vi "LVClass_Camera get Parameter Int.vi"(0 "Camera in":refnum<class "Camera.lvclass">, 7 "parameter_name":string, 11 "error in (no error)":errorcluster) -> (4 "Camera out":refnum<class "Camera.lvclass">, 8 "value":i32, 15 "error out":errorcluster)   [LabVIEW 2020, in "Camera.lvclass"]
doc: "Camera parameter getter for parameter of type E_TYPE_INT.\n\n<B>CameraIn</B> : Camera object.\n<B>CameraOut</B> : Camera object.\n<B>parameter_name</B> : Name of the parameter.\n<B>value</B> : Value of the parameter."
uses:
  Camera.lvclass
  Camera.lvclass/Camera.ctl
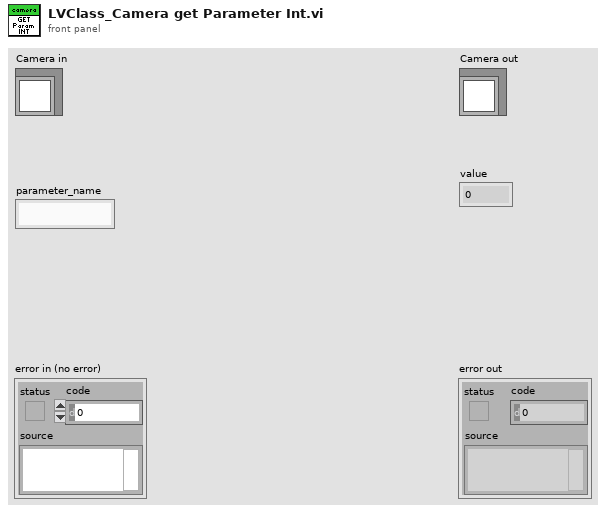
[diagram p1: front panel]
types:
  T1 = typedef "ClassID.ctl" = i64
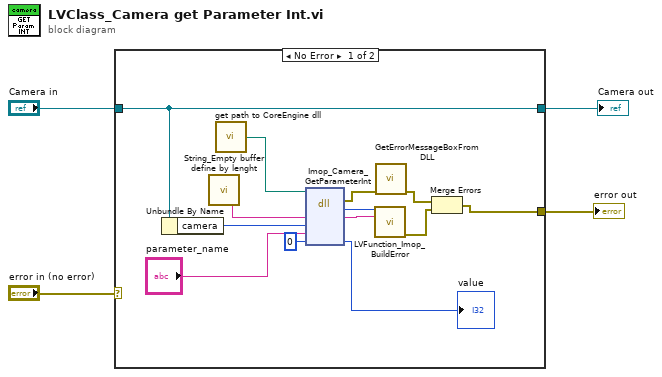
[diagram p0: block diagram]
diagram:
  n1 = case shown="No Error" "error in (no error)" {
    selector: "error in (no error)" -> [_ w19]
    tunnel: [w5 w19] -> w3
    tunnel: [w13 w18] -> w1
    tunnel: "Camera in" -> [w13 w18]
    frame No Error {
      n2 = Unbundle By Name(w13) -> ("camera"=w14:T1)
      n3 = call "String_Empty buffer define by lenght.vi"() -> ("Empty buffer"=w17:string)  [unwired: 1 in]
      n4 = call "get path to CoreEngine dll.vi"() -> ("path to c_interface_vc100.dll"=w12:path)  [unwired: 12 in, 3 out]
      n5 = dll-call lib="D:/2_trunk/Soft_haso/ImOpCoreEngine4_LV2011/DLLs/ImopEngine4_vc100.dll" fn="Imop_Camera_GetParameterInt"(path in=w12, "message"=w17, "camera"=w14, "parameter_name"="parameter_name", "value"=u32 0) -> (error out=w11:errorcluster, "return type"=w16:i32, "message"=w15:string, "value"=→"value":i32)  [unwired: 4 in, 1 out]
      n6 = call "LVFunction_Imop_BuildError.vi"("code"=w16, "String to Prepend to source (\"\")"=w15) -> ("error out"=w6:errorcluster)  [unwired: 13 in]
      n7 = call "GetErrorMessageBoxFromDLL.vi"("error IN"=w11) -> ("error OUT"=w7:errorcluster)  [unwired: 10 in]
      n8 = Merge Errors(w7, w6) -> (w5:errorcluster)
    }
    frame Error {
    }
  }
  "error out" <- w3
  "Camera out" <- w1
